vi "asdfasdf.vi"(7 "path tag":string="prod", 8 "error in":errorcluster, 10 "VIs base path":path=path "/user/pma/PM_app86") -> (0 "error out":errorcluster, 2 "paths with MTAdoc path":path[](array[path]))   [LabVIEW 2010]
panel:
  out "size(s)":i32
  out "Numeric":i32
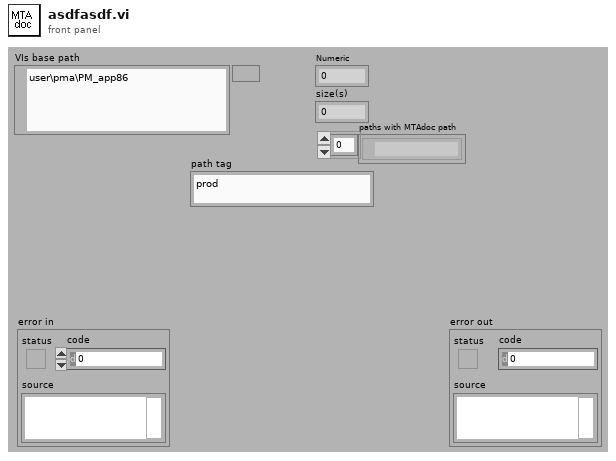
[diagram p1: front panel]
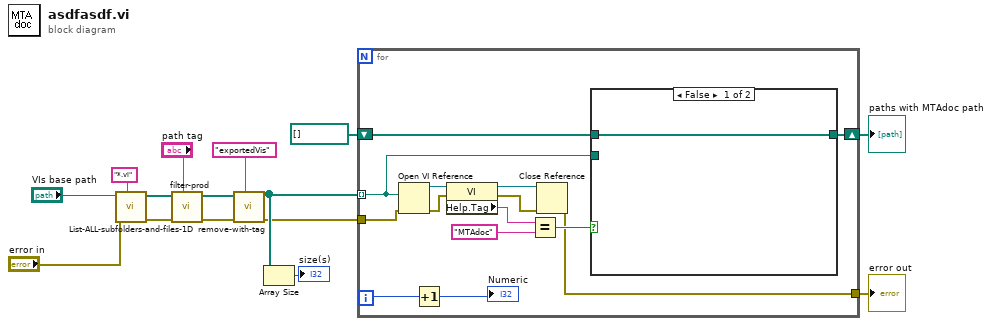
[diagram p0: block diagram]
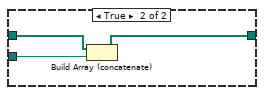
[diagram p2: hidden frame]
diagram:
  n1 = call "List-ALL-subfolders-and-files-1D.vi"("pattern"="*.vi", "error in"="error in", "Top level folder"="VIs base path") -> ("error IO"=w3:errorcluster, "files found"=w12:path[])  [unwired: 7 out]
  n2 = call "filter-prod.vi"("path tag"="path tag", "files found"=w12) -> ("only paths containing tag"=w13:path[])  [unwired: 9 out]
  n3 = call "remove-with-tag.vi"("path tag"="exportedVis", "files found"=w13) -> ("only paths containing tag"=w7:path[])  [unwired: 9 out]
  n4 = Array Size(array=w7) -> (size(s)=→"size(s)":i32)
  n5 = for {
    tunnel: w7 -> [w20] mode=indexing
    shift-right: [w16] -> w4
    shift-left: path[] [] -> [w17]
    tunnel: w3 -> [w15]
    tunnel: [w14] -> w1
    i -> [w19]
    n6 = Open VI Reference(vi path=w20, error in (no error)=w15) -> (vi reference=w22:refnum<vi>, error out=w23:errorcluster)  [unwired: 1 in, 3 out]
    n7 = Increment(x=w19) -> (x+1=→"Numeric":i32)
    n8 = property class="VI"(reference=w22, error in=w23) -> (reference out=w26:refnum<vi>, error out=w27:errorcluster, "Help.Tag"=w24:string)
    n9 = Equal?(x=w24, y="MTAdoc") -> (x = y?=w21:bool)
    n10 = Close Reference(reference=w26, error in (no error)=w27) -> (error out=w14:errorcluster)
    n11 = case shown="False" w21 {
      tunnel: w20 -> [_ w31]
      tunnel: w17 -> [w28 w30]
      tunnel: [w28 w29] -> w16
      frame False {
      }
      frame True {
        n12 = Build Array (concatenate)(w30, w31) -> (w29:path[])
      }
    }
  }
  "paths with MTAdoc path" <- w4
  "error out" <- w1
